vi "Integrate_dPdt.vi"(6 "Measured Current (pA)":dbl[](array[numeric]), 7 "Sample area (mm^2)":dbl, 8 "Averaged?":bool=TRUE, 9 "Temperature array":dbl[](array[numeric]), 10 "Elapsed Time (s)":dbl[](array[numeric]), 11 "dt (s)":dbl) -> (0 "P(T)":cluster{"yi":dbl[], dbl[]}(graph), 2 "Sampled I (pA)":dbl[](array[numeric]) format="%_6g", 3 "Equidistant time":dbl[](array[numeric]))   [LabVIEW 2015]
uses:
  <vilib>/Analysis/baseanly.llb/Mean (DBL).vi
  <vilib>/gmath/NI_Gmath.lvlib
  <vilib>/Analysis/NI_AALBase.lvlib
panel:
  out "P array (uC/m^2)":dbl[](array[numeric])
  out "P array (pC)":dbl[](array[numeric])
  in  "Offset Samples":i32=100
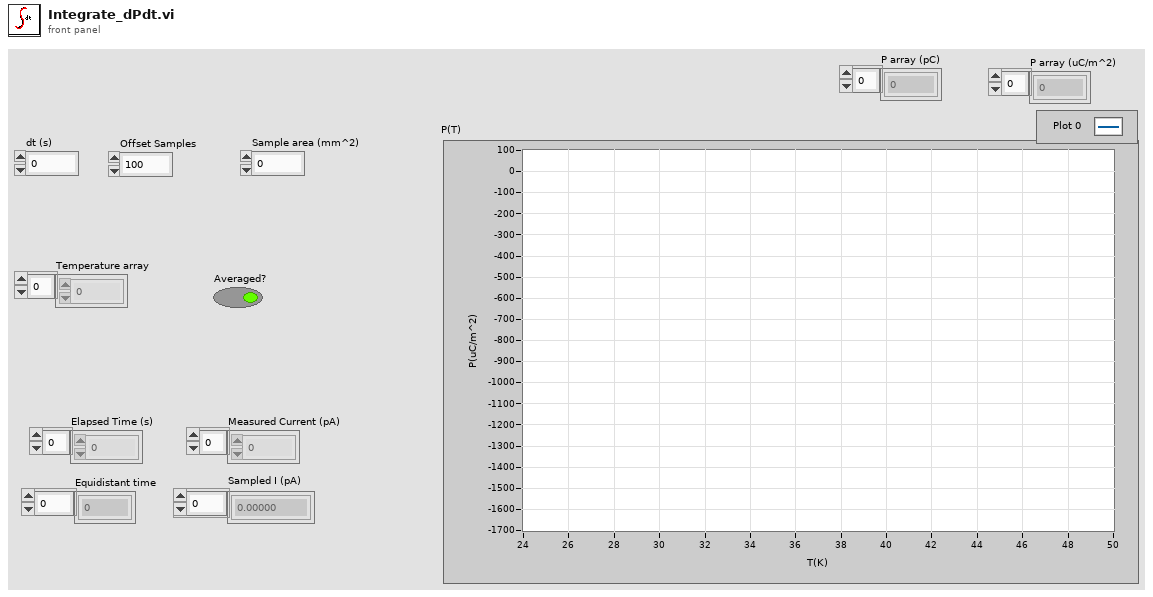
[diagram p1: front panel]
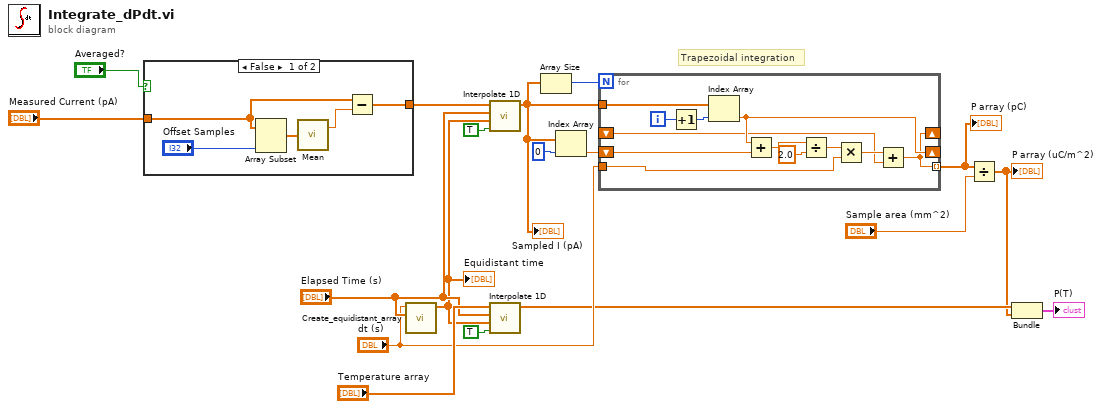
[diagram p0: block diagram]
diagram:
  # "Trapezoidal integration"
  n1 = case shown="False" "Averaged?" {
    tunnel: "Measured Current (pA)" -> [w21 w24]
    tunnel: [w19 w24] -> w7
    frame False {
      n2 = Array Subset(array=w21, length="Offset Samples") -> (w22:dbl[])  [unwired: 1 in]
      n3 = call-poly <vilib>:"Mean.vi"("X"=w22) -> ("mean"=w20:dbl)  [unwired: 1 out]
      n4 = Subtract(x=w21, y=w20) -> (x-y=w19:dbl[])
    }
    frame True {
    }
  }
  n5 = call "Create_equidistant_array.vi"("Elapsed Time (s)"="Elapsed Time (s)", "dt (s)"="dt (s)") -> ("Array"=w14:dbl[])  [unwired: 9 in]
  "Equidistant time" <- w14
  n6 = call <vilib>:"Interpolate 1D.vi"("X is monotonic"=TRUE, "xi"=w14, "X"="Elapsed Time (s)", "Y"=w7) -> ("yi"=w11:dbl[])  [unwired: 5 in, 2 out]
  "Sampled I (pA)" <- w11
  n7 = call <vilib>:"Interpolate 1D.vi"("X is monotonic"=TRUE, "xi"=w14, "X"="Elapsed Time (s)", "Y"="Temperature array") -> ("yi"=w4:dbl[])  [unwired: 5 in, 2 out]
  n8 = Array Size(array=w11) -> (size(s)=w10:i32)
  n9 = Index Array(array=w11, index=0) -> (element=w12:dbl)
  n10 = for {
    N: w10 -> [_]
    tunnel: w11 -> [w35]
    shift-right: [w33] -> _
    shift-left: w12 -> [w32]
    tunnel: "dt (s)" -> [w28]
    shift-right: [w25] -> _
    shift-left: _ -> [w26]
    tunnel: [w25] -> w2 mode=indexing
    i -> [w36]
    n11 = Increment(x=w36) -> (x+1=w34:i32)
    n12 = Index Array(array=w35, index=w34) -> (element=w33:dbl)
    n13 = Add(x=w33, y=w32) -> (x+y=w31:dbl)
    n14 = Divide(x=w31, y=2.0) -> (x/y=w29:dbl)
    n15 = Multiply(x=w29, y=w28) -> (x*y=w27:dbl)
    n16 = Add(x=w27, y=w26) -> (x+y=w25:dbl)
  }
  "P array (pC)" <- w2
  n17 = Divide(x=w2, y="Sample area (mm^2)") -> (x/y=w1:dbl[])
  "P array (uC/m^2)" <- w1
  n18 = Bundle("yi"=w4, w1) -> (→"P(T)":cluster{"yi":dbl[], dbl[]})  [unwired: 1 in]
